vi "Datasheet PIM Last N.vi"(10 "full waveform":dbl[](array[numeric]), 11 "n points":i32) -> (3 "last n pnts waveform":dbl[](array[numeric]))   [LabVIEW 2011]
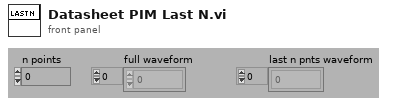
[diagram p1: front panel]
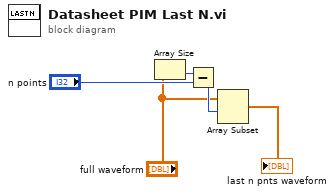
[diagram p0: block diagram]
diagram:
  n1 = Array Size(array="full waveform") -> (size(s)=w3:i32)
  n2 = Subtract(x=w3, y="n points") -> (x-y=w5:i32)
  n3 = Array Subset(array="full waveform", index=w5) -> (→"last n pnts waveform":dbl[])  [unwired: 1 in]
